vi "Measure.vi"(6 "error in (no error)":errorcluster, 9 "Yokogawa WT500 in":refnum<class "Yokogawa WT500.lvclass">) -> (0 "error out":errorcluster, 2 "Array of Measurement":dbl[](array[numeric]), 3 "Yokogawa WT500 out":refnum<class "Yokogawa WT500.lvclass">)   [LabVIEW 2014, in "Generic Power Analyzer.lvlib" / "Yokogawa WT500.lvlib" / "Yokogawa WT500.lvclass"]
uses:
  Yokogawa WT500.lvclass
  <instrlib>/ykwt500/ykwt500.llb/YKWT500 Read Numeric (Normal).vi
  Generic Power Analyzer/Generic Power Analyzer.lvclass
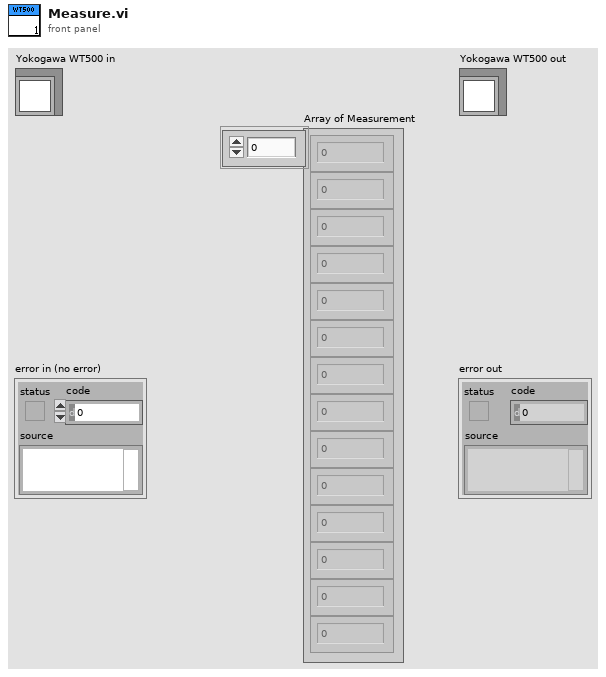
[diagram p1: front panel]
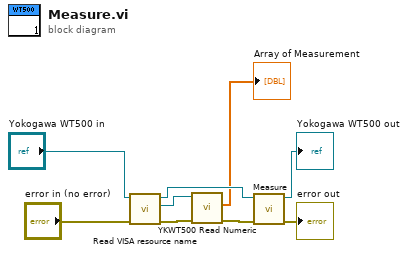
[diagram p0: block diagram]
diagram:
  n1 = call-dynamic "Read VISA resource name.vi"("error in (no error)"="error in (no error)", "Generic Instrument in"="Yokogawa WT500 in") -> ("error out"=w2:errorcluster, "VISA resource name"=w3:refnum<visa-resource-name>, "Generic Instrument out"=w4:refnum<class "Yokogawa WT500.lvclass">)  [unwired: 7 in]
  n2 = call-poly <instrlib>:"YKWT500 Read Numeric.vi"("error in (no error)"=w2, "VISA resource name"=w3) -> ("error out"=w6:errorcluster, "Measurement Value"=→"Array of Measurement":dbl[])  [unwired: 7 in, 1 out]
  n3 = call-parent "Measure.vi"("error in (no error)"=w6, "Generic Power Analyzer in"=w4) -> ("error out"=→"error out":errorcluster, "Generic Power Analyzer out"=→"Yokogawa WT500 out":refnum<class "Yokogawa WT500.lvclass">)  [unwired: 5 in, 1 out]
